vi "Sensor_Reads.vi"() -> ()   [LabVIEW 2019]
uses:
  <vilib>/Rock Robotics/WPI/ThirdParty/Phoenix-LabVIEW/Motor Controller/Get/CTRE_Phoenix_MotorController_GetPulseWidthAll.vi
  Globals/Drive_Globals.vi
  <vilib>/Rock Robotics/WPI/ThirdParty/Phoenix-LabVIEW/Motor Controller/Get/CTRE_Phoenix_MotorController_GetQuadratureData.vi
  Globals/Sensor_Values.vi
  <vilib>/Rock Robotics/WPI/ThirdParty/Phoenix-LabVIEW/Pigeon IMU/CTRE_PigeonIMU_GetYPR.vi
  <vilib>/Rock Robotics/Network Tables/NT Read Number.vi
  M14 Hardware/Magazine/Magazine_Hardware_Globals.vi
panel:
  out "BL mod":i32=2998
  out "BR mod":i32=373
  out "FL mod":i32=1419
  out "FR mod":i32=3907
  out "deltat":u32=21
  out "Back_left":i32=15286
  out "Back_Right":i32=8565
  out "front right":i32=16195
  out "Front_left":i32=9611
  in  "Back_Right_Zero":i32=3179
  in  "Back_Left_Zero":i32=57
  in  "Front_Left_Zero":i32=227
  in  "Front_Right_Zero":i32=759
  # "e"
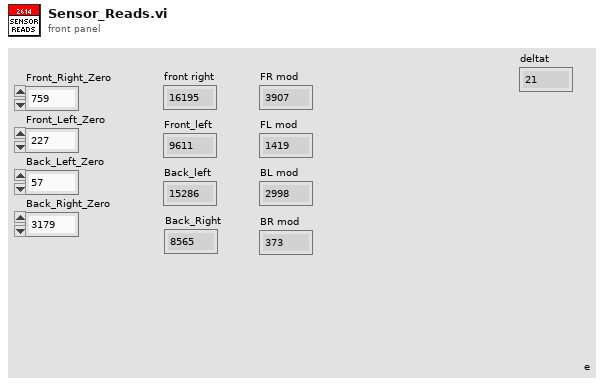
[diagram p1: front panel]
types:
  T1 = typedef "WPI_MotorControlDeviceRef.ctl" = cluster{"DeviceStatus":errorcluster, "Type":T2, "PWM":cluster{"PWM Channel":T3, "DeadBand":T4}, "CAN":cluster{"Device Number":u8, "SetOutput VI Ref":variant, "GetOutput VI Ref":variant, "Enable VI Ref":variant, "Disable VI Ref":variant, "Data":variant}, "Invert":bool, "DIO PWM":cluster{"PWM \"Enable\" Channel":T3, "DIOChannel":T5, "PWM Rate":dbl}}
  T2 = typedef "WPI_MotorControlType.ctl" = enum16{"PWM", "CAN", "DIO PWM"}
  T3 = typedef "FPGA_DIOPWMChannel.ctl" = enum8{"PWM 0", "PWM 1", "PWM 2", "PWM 3", "PWM 4", "PWM 5", "PWM 6", "PWM 7", "PWM 8", "PWM 9", "PWM MXP 0", "PWM MXP 1", "PWM MXP 2", "PWM MXP 3", "PWM MXP 4", "PWM MXP 5", "PWM MXP 6", "PWM MXP 7", "PWM MXP 8", "PWM MXP 9", "Invalid"}
  T4 = typedef "WPI_PWMDeadband.ctl" = cluster{"Name":string, "maxPositivePwm":i32, "minPositivePwm":i32, "centerPwm":i32, "maxNegativePwm":i32, "minNegativePwm":i32, "angularRange":u16}
  T5 = typedef "FPGA_DIOChannel.ctl" = enum8{"DIO 0", "DIO 1", "DIO 2", "DIO 3", "DIO 4", "DIO 5", "DIO 6", "DIO 7", "DIO 8", "DIO 9", "DIO MXP 0", "DIO MXP 1", "DIO MXP 2", "DIO MXP 3", "DIO MXP 4", "DIO MXP 5", "DIO MXP 6", "DIO MXP 7", "DIO MXP 8", "DIO MXP 9", "DIO MXP 10", "DIO MXP 11", "DIO MXP 12", "DIO MXP 13", "DIO MXP 14", "DIO MXP 15", "SPI Port CS1", "SPI Port CS2", "SPI Port CS3", "SPI Port MISO", "SPI Port MOSI", "Invalid"}
  T6 = typedef "CTRE_PigeonIMU_DeviceRef.ctl" = cluster{"DeviceStatus":errorcluster, "Device Number":u8, "Type":T7, "Device ID":u32, "Handle":u64, "UsageFrame":u32, "Library Path":path}
  T7 = typedef "CTRE_PigeonIMU_ConnectionType.ctl" = u32
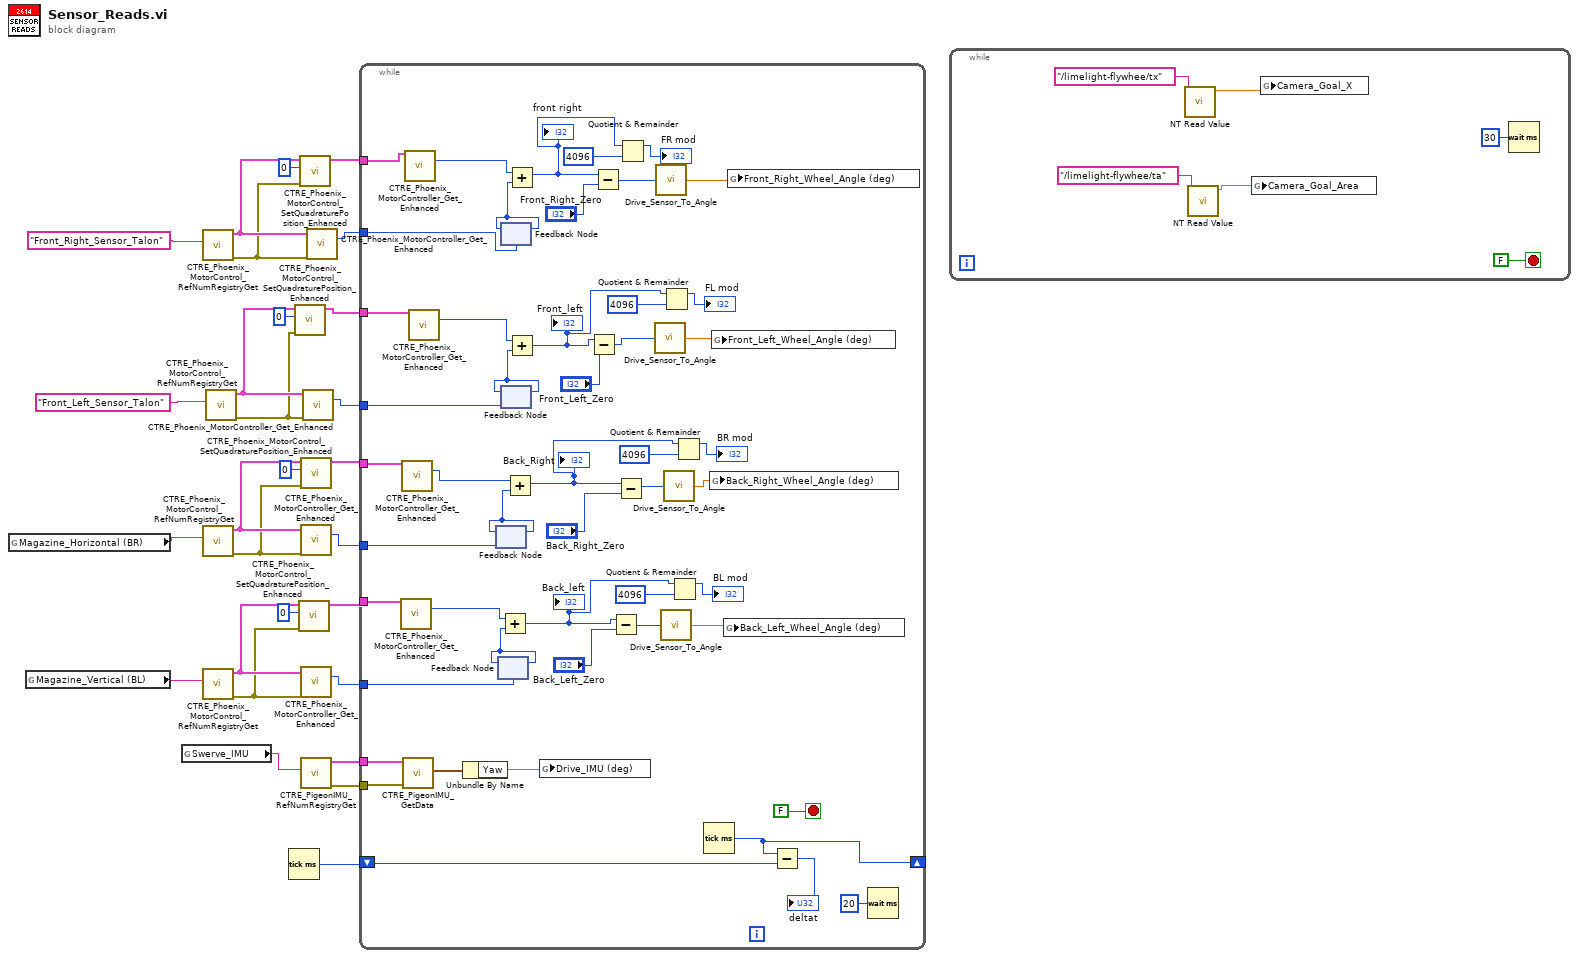
[diagram p0: block diagram]
diagram:
  n1 = global read "Magazine_Hardware_Globals.vi" "Magazine_Horizontal (BR)"() -> (w2:string)
  n2 = global read "Magazine_Hardware_Globals.vi" "Magazine_Vertical (BL)"() -> (w1:string)
  n3 = global read "Drive_Globals.vi" "Swerve_IMU"() -> (w26:string)
  n4 = call <vilib>:"CTRE_Phoenix_MotorControl_RefNumRegistryGet.vi"("refnum name"="Front_Right_Sensor_Talon") -> ("error out"=w15:errorcluster, "PhoenixMotorControlDevRef"=w18:T1)  [unwired: 9 in]
  n5 = call <vilib>:"CTRE_Phoenix_MotorControl_RefNumRegistryGet.vi"("refnum name"=w2) -> ("error out"=w7:errorcluster, "PhoenixMotorControlDevRef"=w12:T1)  [unwired: 9 in]
  n6 = call <vilib>:"CTRE_Phoenix_MotorControl_RefNumRegistryGet.vi"("refnum name"=w1) -> ("error out"=w8:errorcluster, "PhoenixMotorControlDevRef"=w9:T1)  [unwired: 9 in]
  n7 = call <vilib>:"CTRE_Phoenix_MotorControl_RefNumRegistryGet.vi"("refnum name"="Front_Left_Sensor_Talon") -> ("error out"=w6:errorcluster, "PhoenixMotorControlDevRef"=w13:T1)  [unwired: 9 in]
  n8 = Tick Count (ms)() -> (millisecond timer value=w19:u32)
  n9 = call <vilib>:"CTRE_Phoenix_MotorControl_SetQuadraturePosition_Enhanced.vi"("error in (no error)"=w6, "New Position"=0, "PhoenixMotorControlDevRef"=w13) -> ("PhoenixMotorControlDevRef"=w14:T1)  [unwired: 7 in, 1 out]
  n10 = call <vilib>:"CTRE_Phoenix_MotorControl_SetQuadraturePosition_Enhanced.vi"("error in (no error)"=w8, "New Position"=0, "PhoenixMotorControlDevRef"=w9) -> ("PhoenixMotorControlDevRef"=w10:T1)  [unwired: 7 in, 1 out]
  n11 = call <vilib>:"CTRE_Phoenix_MotorControl_SetQuadraturePosition_Enhanced.vi"("error in (no error)"=w15, "New Position"=0, "PhoenixMotorControlDevRef"=w18) -> ("PhoenixMotorControlDevRef"=w17:T1)  [unwired: 7 in, 1 out]
  n12 = call <vilib>:"CTRE_Phoenix_MotorControl_SetQuadraturePosition_Enhanced.vi"("error in (no error)"=w7, "New Position"=0, "PhoenixMotorControlDevRef"=w12) -> ("PhoenixMotorControlDevRef"=w11:T1)  [unwired: 7 in, 1 out]
  n13 = call-poly <vilib>:"CTRE_Phoenix_MotorController_Get_Enhanced.vi"("PhoenixMotorControlDevRef"=w12, "error in"=w7) -> ("Pulse Width Position"=w23:i32)  [unwired: 8 in, 5 out]
  n14 = call-poly <vilib>:"CTRE_Phoenix_MotorController_Get_Enhanced.vi"("PhoenixMotorControlDevRef"=w9, "error in"=w8) -> ("Pulse Width Position"=w20:i32)  [unwired: 8 in, 5 out]
  n15 = call <vilib>:"CTRE_PigeonIMU_RefNumRegistryGet.vi"("refnum name"=w26) -> ("error out"=w27:errorcluster, "PigeonIMUDevRef"=w28:T6)  [unwired: 9 in]
  n16 = call-poly <vilib>:"CTRE_Phoenix_MotorController_Get_Enhanced.vi"("PhoenixMotorControlDevRef"=w13, "error in"=w6) -> ("Pulse Width Position"=w22:i32)  [unwired: 8 in, 5 out]
  n17 = call-poly <vilib>:"CTRE_Phoenix_MotorController_Get_Enhanced.vi"("PhoenixMotorControlDevRef"=w18, "error in"=w15) -> ("Pulse Width Position"=w21:i32)  [unwired: 8 in, 5 out]
  n18 = while {
    tunnel: w28 -> [w75]
    tunnel: w27 -> [w72]
    tunnel: w17 -> [w51]
    tunnel: w14 -> [w50]
    tunnel: w11 -> [w49]
    tunnel: w10 -> [w48]
    tunnel: w23 -> [w47]
    tunnel: w22 -> [w46]
    tunnel: w21 -> [w45]
    tunnel: w20 -> [w44]
    shift-right: [w42] -> _
    shift-left: w19 -> [w43]
    stop <- FALSE stop-if-true
    n19 = call-poly <vilib>:"CTRE_Phoenix_MotorController_Get_Enhanced.vi"("PhoenixMotorControlDevRef"=w48) -> ("Quadrature Position"=w55:i32)  [unwired: 11 in, 3 out]
    n20 = call-poly <vilib>:"CTRE_Phoenix_MotorController_Get_Enhanced.vi"("PhoenixMotorControlDevRef"=w49) -> ("Quadrature Position"=w61:i32)  [unwired: 11 in, 3 out]
    n21 = call-poly <vilib>:"CTRE_PigeonIMU_GetData.vi"("error in (no error)"=w72, "PigeonIMUDevRef"=w75) -> ("Yaw Pitch Roll"=w74:cluster{"Yaw":dbl, "Pitch":dbl, "Roll":dbl})  [unwired: 7 in, 2 out]
    n22 = call-poly <vilib>:"CTRE_Phoenix_MotorController_Get_Enhanced.vi"("PhoenixMotorControlDevRef"=w51) -> ("Quadrature Position"=w71:i32)  [unwired: 11 in, 3 out]
    n23 = call-poly <vilib>:"CTRE_Phoenix_MotorController_Get_Enhanced.vi"("PhoenixMotorControlDevRef"=w50) -> ("Quadrature Position"=w66:i32)  [unwired: 11 in, 3 out]
    n24 = Unbundle By Name(w74) -> ("Yaw"=w73:dbl)
    n25 = feedback #1(w47) -> (w60:i32)
    n26 = feedback-in #1(w60) -> ()
    n27 = feedback #2(w44) -> (w56:i32)
    n28 = feedback-in #2(w56) -> ()
    n29 = Add(x=w55, y=w56) -> (x+y=w35:i32)
    "Back_left" <- w35
    n30 = feedback #3(w45) -> (w70:i32)
    n31 = feedback-in #3(w70) -> ()
    n32 = feedback #4(w46) -> (w65:i32)
    n33 = feedback-in #4(w65) -> ()
    n34 = Add(x=w61, y=w60) -> (x+y=w34:i32)
    "Back_Right" <- w34
    n35 = Add(x=w71, y=w70) -> (x+y=w40:i32)
    "front right" <- w40
    n36 = Add(x=w66, y=w65) -> (x+y=w33:i32)
    "Front_left" <- w33
    n37 = global write "Sensor_Values.vi" "Drive_IMU (deg)"(w73) -> ()
    n38 = Subtract(x=w33, y="Front_Left_Zero") -> (x-y=w63:i32)
    n39 = Subtract(x=w40, y="Front_Right_Zero") -> (x-y=w67:i32)
    n40 = Subtract(x=w35, y="Back_Left_Zero") -> (x-y=w53:i32)
    n41 = Subtract(x=w34, y="Back_Right_Zero") -> (x-y=w57:i32)
    n42 = Quotient & Remainder(x=w40, y=4096 ("x+y")) -> (x-y*floor(x/y)=→"FR mod":i32)  [unwired: 1 out]
    n43 = call "Drive_Sensor_To_Angle.vi"("Position (Raw Sensor Units)"=w63) -> ("Numeric"=w62:dbl)
    n44 = call "Drive_Sensor_To_Angle.vi"("Position (Raw Sensor Units)"=w67) -> ("Numeric"=w68:dbl)
    n45 = call "Drive_Sensor_To_Angle.vi"("Position (Raw Sensor Units)"=w53) -> ("Numeric"=w52:dbl)
    n46 = Quotient & Remainder(x=w33, y=4096 ("x+y")) -> (x-y*floor(x/y)=→"FL mod":i32)  [unwired: 1 out]
    n47 = call "Drive_Sensor_To_Angle.vi"("Position (Raw Sensor Units)"=w57) -> ("Numeric"=w58:dbl)
    n48 = Quotient & Remainder(x=w35, y=4096 ("x+y")) -> (x-y*floor(x/y)=→"BL mod":i32)  [unwired: 1 out]
    n49 = Quotient & Remainder(x=w34, y=4096 ("x+y")) -> (x-y*floor(x/y)=→"BR mod":i32)  [unwired: 1 out]
    n50 = Tick Count (ms)() -> (millisecond timer value=w42:u32)
    n51 = global write "Sensor_Values.vi" "Back_Right_Wheel_Angle (deg)"(w58) -> ()
    n52 = global write "Sensor_Values.vi" "Front_Left_Wheel_Angle (deg)"(w62) -> ()
    n53 = global write "Sensor_Values.vi" "Back_Left_Wheel_Angle (deg)"(w52) -> ()
    n54 = global write "Sensor_Values.vi" "Front_Right_Wheel_Angle (deg)"(w68) -> ()
    n55 = Subtract(x=w42, y=w43) -> (x-y=→"deltat":u32)
    n56 = Wait (ms)(milliseconds to wait=u32 20) -> ()  [unwired: 1 out]
  }
  n57 = while {
    stop <- FALSE stop-if-true
    n58 = call-poly <vilib>:"NT Read Value.vi"("Name"="/limelight-flywhee/tx") -> ("Numeric"=w83:dbl)  [unwired: 9 in, 1 out]
    n59 = call-poly <vilib>:"NT Read Value.vi"("Name"="/limelight-flywhee/ta") -> ("Numeric"=w82:dbl)  [unwired: 9 in, 1 out]
    n60 = global write "Sensor_Values.vi" "Camera_Goal_Area"(w82) -> ()
    n61 = global write "Sensor_Values.vi" "Camera_Goal_X"(w83) -> ()
    n62 = Wait (ms)(milliseconds to wait=u32 30) -> ()  [unwired: 1 out]
  }
